vi "Saving_Warnings(SubVI).vi"(7 "Warnings bool array":bool[](array[boolean]), 8 "Reset":bool, 11 "W In":string[][](array[string])) -> (3 "W Out":string[][](array[string]))   [LabVIEW 2022 SP3]
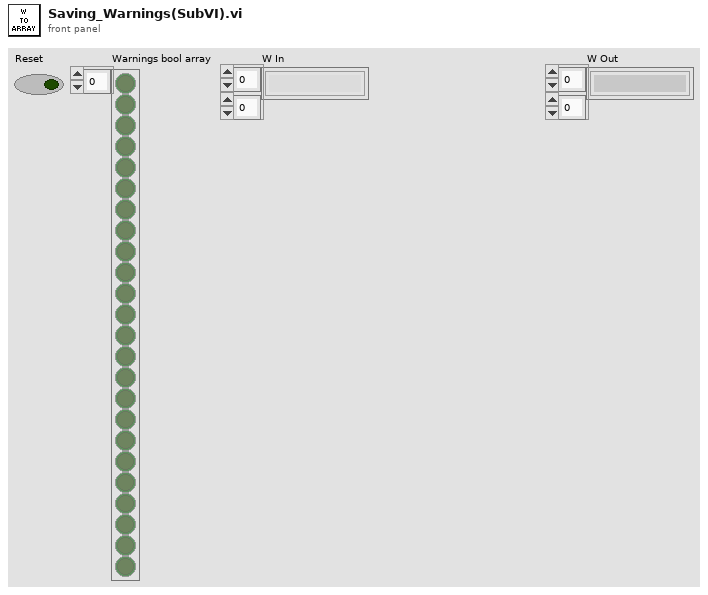
[diagram p1: front panel]
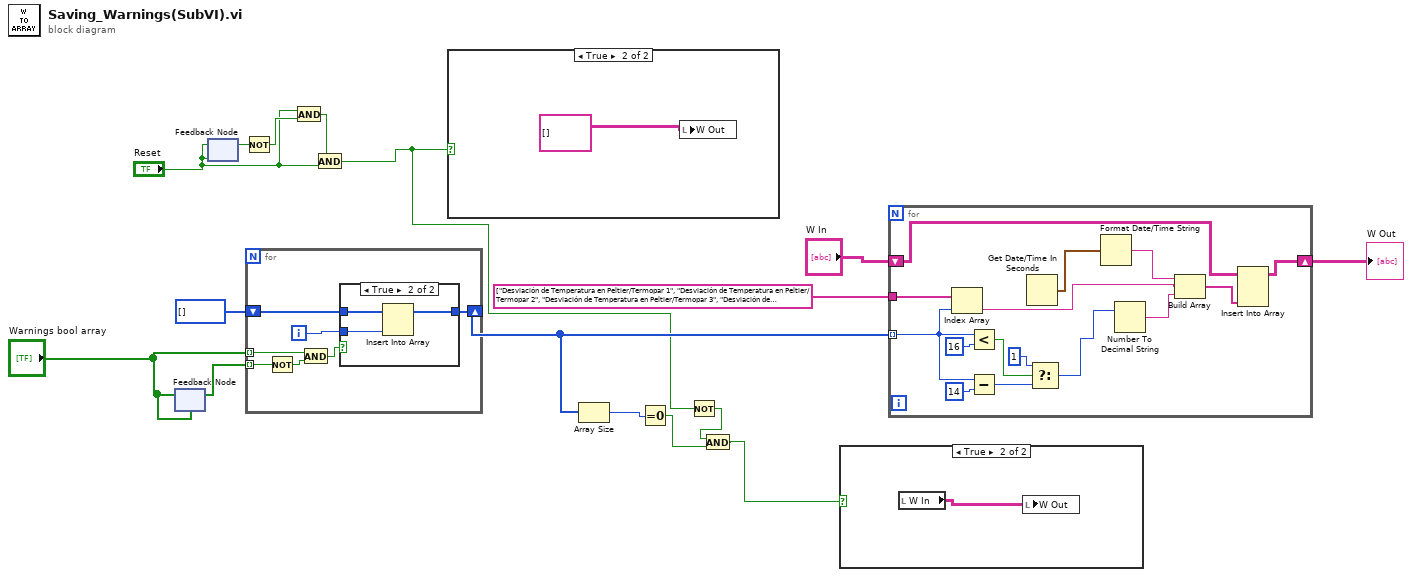
[diagram p0: block diagram]
diagram:
  n1 = feedback #1("Warnings bool array") -> (w13:bool[])
  n2 = feedback-in #1("Warnings bool array") -> ()
  n3 = feedback #2("Reset") -> (w9:bool)
  n4 = feedback-in #2("Reset") -> ()
  n5 = Not(x=w9) -> (.not. x?=w10:bool)
  n6 = for {
    tunnel: w13 -> [w23] mode=indexing
    tunnel: "Warnings bool array" -> [w21] mode=indexing
    shift-right: [w17] -> w12
    shift-left: i32[] [] -> [w20]
    i -> [w19]
    n7 = Not(x=w23) -> (.not. x?=w22:bool)
    n8 = And(x=w21, y=w22) -> (x .and. y?=w18:bool)
    n9 = case shown="True" w18 {
      tunnel: w20 -> [w24 w27]
      tunnel: w19 -> [_ w25]
      tunnel: [w24 w26] -> w17
      frame False {
      }
      frame True {
        n10 = Insert Into Array(array=w27, new element=w25) -> (w26:i32[])  [unwired: 1 in]
      }
    }
  }
  n11 = And(x="Reset", y=w10) -> (x .and. y?=w8:bool)
  n12 = And(x=w8, y="Reset") -> (x .and. y?=w4:bool)
  n13 = case shown="True" w4 {
    frame False {
    }
    frame True {
      n14 = local write "W Out"(string[][] [] ("W Out")) -> ()
    }
  }
  n15 = Array Size(array=w12) -> (size(s)=w11:i32)
  n16 = Equal To 0?(x=w11) -> (x = 0?=w6:bool)
  n17 = Not(x=w4) -> (.not. x?=w5:bool)
  n18 = And(x=w5, y=w6) -> (x .and. y?=w3:bool)
  n19 = case shown="True" w3 {
    frame False {
    }
    frame True {
      n20 = local read "W In"() -> (w29:string[][])
      n21 = local write "W Out"(w29) -> ()
    }
  }
  n22 = for {
    tunnel: w12 -> [w38] mode=indexing
    tunnel: string[] ["Desviación de Temperatura en Peltier/Termopar 1", "Desviación de Temperatura en Peltier/Termopar 2", "Desviación de Temperatura en Peltier/Termopar 3", "Desviación de Temperatura en Peltier/Termopar 4", "Desviación de Temperatura en Peltier/Termopar 5", "Desviación de Temperatura en Peltier/Termopar 6", "Desviación de Temperatura en Peltier/Termopar 7", "Desviación de Temperatura en Peltier/Termopar 8", "Desviación de Temperatura en Peltier/Termopar 9", "Desviación de Temperatura en Peltier/Termopar 10", "Desviación de Temperatura en Peltier/Termopar 11", "Desviación de Temperatura en Peltier/Termopar 12", "Desviación de Temperatura en Peltier/Termopar 13", "Desviación de Temperatura en Peltier/Termopar 14", "Desviación de Temperatura en Peltier/Termopar 15", "Desviación de Temperatura en Peltier/Termopar 16", "Desviación de Temperatura en la CC.", "Disparo del valor LEL (%). AMBIENTE EXPLOSIVO", "Valor anómalo de O2(%)"] -> [w44]
    shift-right: [w30] -> w2
    shift-left: "W In" -> [w31]
    n23 = Index Array(array=w44, index=w38) -> (element=w35:string)
    n24 = Less?(x=w38, y=16) -> (x < y?=w42:bool)
    n25 = Subtract(x=w38, y=14) -> (x-y=w39:i32)
    n26 = Get Date/Time In Seconds() -> (seconds since 1Jan1904=w34:timestamp)
    n27 = Select(t=1, s=w42, f=w39) -> (s? t:f=w37:i32)
    n28 = Format Date/Time String(seconds (now)=w34) -> (date/time string=w33:string)  [unwired: 2 in]
    n29 = Number To Decimal String(number=w37) -> (decimal integer string=w36:string)  [unwired: 1 in]
    n30 = Build Array(w33, w35, w36) -> (w32:string[])
    n31 = Insert Into Array(array=w31, new element=w32) -> (w30:string[][])  [unwired: 2 in]
  }
  "W Out" <- w2
